vi "Img Update Frame Image.vi"(8 "error in (no error)":errorcluster, 11 "LF2R IDE in":refnum<class "Main Panel.lvclass">) -> (0 "error out":errorcluster, 3 "LF2R IDE out":refnum<class "Main Panel.lvclass">)   [LabVIEW 2018, in "Main Panel.lvlib" / "Main Panel.lvclass"]
uses:
  Main Panel.lvclass
  Main Panel.lvclass/Main Panel.ctl
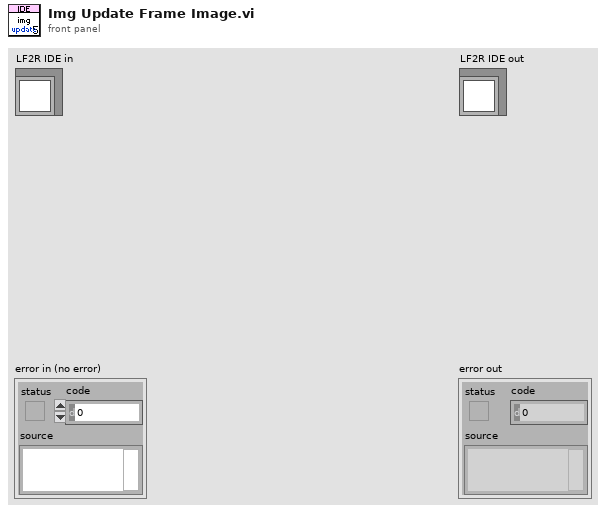
[diagram p1: front panel]
types:
  T1 = typedef "imagedata.ctl" = cluster{"image type":i32, "image depth":i32, "image":u8[], "mask":u8[], "colors":u32[], "Rectangle":cluster{"left":i16, "top":i16, "right":i16, "bottom":i16}}
  T2 = typedef "Image Json Parser.lvclass/Img Json Data.ctl" = cluster{"frames":T3[], "meta":T4}
  T3 = typedef "Image Json Parser.lvclass/Img Json Frames.ctl" = cluster{"frame":cluster{"x":i32, "y":i32, "w":i32, "h":i32}, "rotated":bool, "trimmed":bool, "spriteSourceSize":cluster{"x":i32, "y":i32, "w":i32, "h":i32}, "sourceSize":cluster{"w":i32, "h":i32}}
  T4 = typedef "Image Json Parser.lvclass/Img Json Meta.ctl" = cluster{"app":string, "version":string, "image":string, "format":string, "size":cluster{"w":i32, "h":i32}, "scale":string}
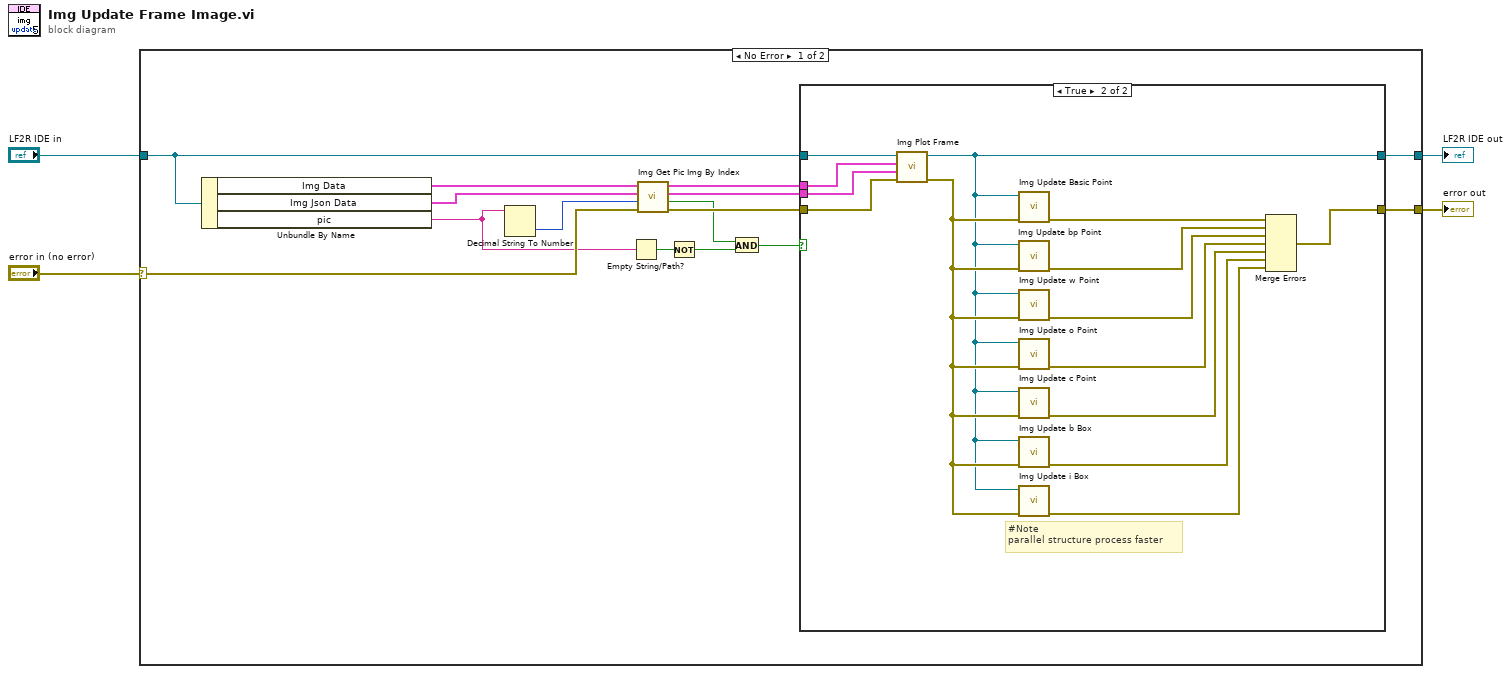
[diagram p0: block diagram]
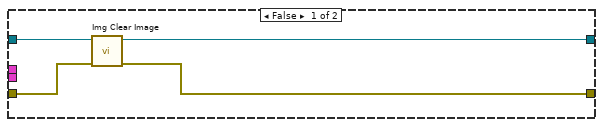
[diagram p2: hidden frame]
diagram:
  n1 = case shown="No Error" "error in (no error)" {
    selector: "error in (no error)" -> [w17 w39]
    tunnel: [w13 w39] -> w3
    tunnel: [w5 w38] -> w1
    tunnel: "LF2R IDE in" -> [w6 w38]
    frame No Error {
      n2 = Unbundle By Name(w6) -> ("Img Data"=w19:cluster{"image data":T1, "bitmap":u32[][]}[], "Img Json Data"=w18:T2[], "pic"=w11:string)
      n3 = Decimal String To Number(string=w11) -> (number=w12:i32)  [unwired: 2 in, 1 out]
      n4 = Empty String/Path?(string/path=w11) -> (empty?=w10:bool)
      n5 = call "Img Get Pic Img By Index.vi"("error in (no error)"=w17, "Pic Num"=w12, "Img Json Data"=w18, "Img Data"=w19) -> ("error out"=w14:errorcluster, "Found?"=w8:bool, "frames"=w16:T3, "Img Data Indexed"=w15:cluster{"image data":T1, "bitmap":u32[][]})  [unwired: 4 in]
      n6 = Not(x=w10) -> (.not. x?=w9:bool)
      n7 = And(x=w8, y=w9) -> (x .and. y?=w7:bool)
      n8 = case shown="True" w7 {
        tunnel: w16 -> [_ w35]
        tunnel: w15 -> [_ w36]
        tunnel: w14 -> [w22 w34]
        tunnel: [w21 w24] -> w13
        tunnel: w6 -> [w23 w37]
        tunnel: [w20 w32] -> w5
        frame False {
          n9 = call "Img Clear Image.vi"("error in (no error)"=w22, "LF2R IDE in"=w23) -> ("error out"=w21:errorcluster, "LF2R IDE out"=w20:refnum<class "Main Panel.lvclass">)  [unwired: 8 in]
        }
        frame True {
          # "#Note\nparallel structure process faster"
          n10 = call "Img Plot Frame.vi"("error in (no error)"=w34, "frames"=w35, "Img Data indexed"=w36, "LF2R IDE in"=w37) -> ("error out"=w33:errorcluster, "LF2R IDE out"=w32:refnum<class "Main Panel.lvclass">)  [unwired: 6 in]
          n11 = call "Img Update Basic Point.vi"("error in (no error)"=w33, "LF2R IDE in"=w32) -> ("error out"=w31:errorcluster)  [unwired: 8 in, 1 out]
          n12 = call "Img Update bp Point.vi"("error in (no error)"=w33, "LF2R IDE in"=w32) -> ("error out"=w30:errorcluster)  [unwired: 8 in, 1 out]
          n13 = call "Img Update w Point.vi"("error in (no error)"=w33, "LF2R IDE in"=w32) -> ("error out"=w29:errorcluster)  [unwired: 8 in, 1 out]
          n14 = call "Img Update o Point.vi"("error in (no error)"=w33, "LF2R IDE in"=w32) -> ("error out"=w28:errorcluster)  [unwired: 8 in, 1 out]
          n15 = call "Img Update c Point.vi"("error in (no error)"=w33, "LF2R IDE in"=w32) -> ("error out"=w27:errorcluster)  [unwired: 8 in, 1 out]
          n16 = call "Img Update b Box.vi"("error in (no error)"=w33, "LF2R IDE in"=w32) -> ("error out"=w26:errorcluster)  [unwired: 8 in, 1 out]
          n17 = call "Img Update i Box.vi"("error in (no error)"=w33, "LF2R IDE in"=w32) -> ("error out"=w25:errorcluster)  [unwired: 8 in, 1 out]
          n18 = Merge Errors(w31, w30, w29, w28, w27, w26, w25) -> (w24:errorcluster)
        }
      }
    }
    frame Error {
    }
  }
  "error out" <- w3
  "LF2R IDE out" <- w1
